vi "Phi-initial.vi"() -> ()   [LabVIEW 2020]
panel:
  out "Phi-Mars":dbl
  out "Phi-Venus":dbl
  out "Phi-Earth":dbl
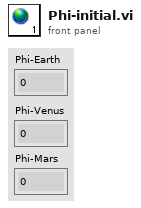
[diagram p1: front panel]
diagram:
